vi "Emballage_BDD_synchroniser_Param.vi"(8 "error in (no error)":errorcluster caption="entrée d'erreur (pas d'erreur)", 11 "Refnum Ch":refnum<vi>) -> (0 "error out":errorcluster caption="sortie d'erreur")   [LabVIEW 2020]
uses:
  Modules/FS/60_FS_Controles/60_FS_SetGet.ctl
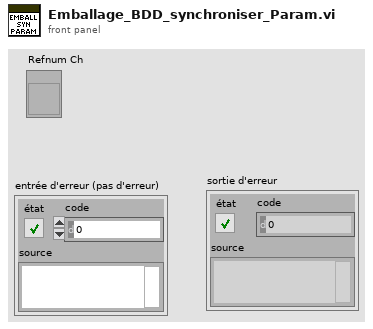
[diagram p1: front panel]
types:
  T1 = typedef "60_FS_SetGet.ctl" = enum16{"set", "get"}
  T2 = typedef "60_FS_CLT_Chemins.ctl" = cluster{"Racine_local":path, "Racine_reseau":path, "Racine_Support_Application":path, "Fichier_Journalisation":path, "Connexion_BDD_VSX":path, "Connexion_BDD_PLZ":path}
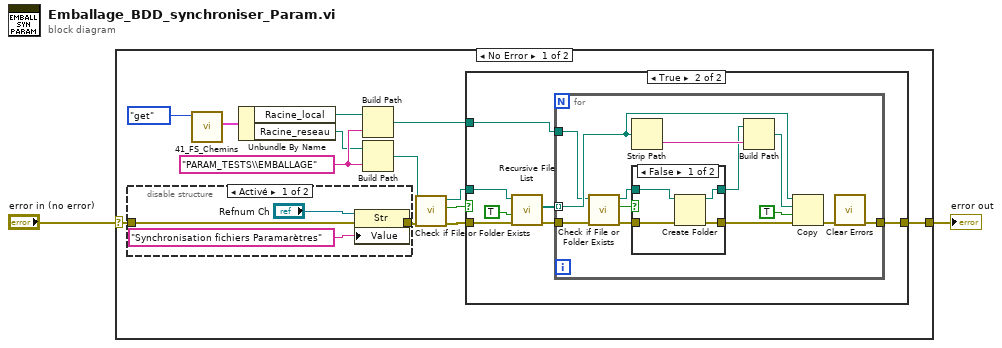
[diagram p0: block diagram]
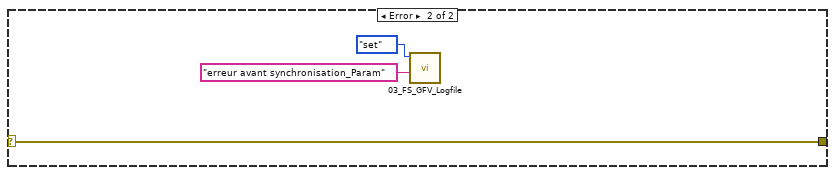
[diagram p5: hidden frame]
diagram:
  n1 = case shown="No Error" "error in (no error)" {
    selector: "error in (no error)" -> [w4 w50]
    tunnel: [w3 w50] -> w1
    frame No Error {
      w9 = "PARAM_TESTS\\EMBALLAGE" ("nom ou chemin relatif")
      n2 = disable-structure shown="Activé" {
        disable-tunnel: [w17 w20] -> w5
        disable-tunnel: w4 -> [w16 w20]
        frame Enabled {
          n3 = property class="Str"(reference="Refnum Ch", error in=w16, "Value"="Synchronisation fichiers Paramarètres" ("Valeur")) -> (error out=w17:errorcluster)  [unwired: 1 out]
        }
        frame Disabled {
        }
      }
      n4 = call "41_FS_Chemins.vi"("SetGet"=60_FS_SetGet."get") -> ("CLT_Chemins_out"=w6:T2)  [unwired: 9 in, 1 out]
      n5 = Unbundle By Name(w6) -> ("Racine_local"=w10:path, "Racine_reseau"=w8:path)
      n6 = Build Path(base path=w10, name or relative path=w9) -> (appended path=w11:path)
      n7 = Build Path(base path=w8, name or relative path=w9) -> (appended path=w13:path)
      n8 = call <vilib>:"Check if File or Folder Exists.vi"("error in (no error)"=w5, "path"=w13) -> ("error out"=w12:errorcluster, "file or folder exists?"=w15:bool, "dup path"=w14:path)  [unwired: 7 in]
      n9 = case shown="True" w15 {
        tunnel: w14 -> [_ w26]
        tunnel: w11 -> [_ w25]
        tunnel: w12 -> [w21 w24]
        tunnel: [w21 w22] -> w3
        frame False {
        }
        frame True {
          n10 = call <vilib>:"Recursive File List.vi"("error in (no error)"=w24, "Continue Recursing on Error? (F)"=TRUE, "Folder Path"=w26) -> ("error out"=w23:errorcluster, "All Files in Dir"=w27:path[])  [unwired: 4 in, 3 out]
          n11 = for {
            tunnel: w27 -> [w38] mode=indexing
            tunnel: w25 -> [w33]
            tunnel: w23 -> [w32]
            tunnel: [w29] -> w22
            n12 = call <vilib>:"Check if File or Folder Exists.vi"("error in (no error)"=w32, "path"=w33) -> ("error out"=w31:errorcluster, "file or folder exists?"=w36:bool, "dup path"=w35:path)  [unwired: 7 in]
            n13 = Strip Path(path=w38) -> (name=w37:string)  [unwired: 1 out]
            n14 = case shown="False" w36 {
              tunnel: w35 -> [w45 w47]
              tunnel: [w44 w47] -> w34
              tunnel: w31 -> [w43 w46]
              tunnel: [w42 w46] -> w30
              frame False {
                n15 = Create Folder(path (use dialog)=w45, error in=w43) -> (created path=w44:path, error out=w42:errorcluster)  [unwired: 1 in, 1 out]
              }
              frame True {
              }
            }
            n16 = Build Path(base path=w34, name or relative path=w37) -> (appended path=w39:path)
            n17 = Copy(8:w30, 9:TRUE ("écraser (F)"), 10:w39, 11:w38) -> (0:w40:errorcluster)  [unwired: 1 in, 2 out]
            n18 = call <vilib>:"Clear Errors.vi"("error in (no error)"=w40) -> ("error out"=w29:errorcluster)  [unwired: 5 in, 1 out]
          }
        }
      }
    }
    frame Error {
      n19 = call "03_FS_GFV_Logfile.vi"("Chaîne"="erreur avant synchronisation_Param", "States"=60_FS_SetGet."set") -> ()  [unwired: 8 in, 2 out]
    }
  }
  "error out" <- w1
